vi "RS_Flip_Flop.vi"(3 "error in (no error)":errorcluster, 4 "Set":bool, 5 "Reset":bool) -> (0 "error out":errorcluster, 1 "Qnot":bool, 2 "Q":bool)   [LabVIEW 2018]
doc: "Set / Reset Flip Flop.\nR=0, S=0, Q=No change\nR=0, S=0, Q=1\nR=1, S=0, Q=0\nR=1, S=1, Q=invalid (will give an error)\n\nwritten by David Huff, DISTek Integration \n(www.distek.com)"
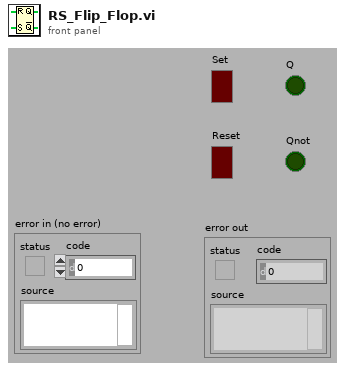
[diagram p1: front panel]
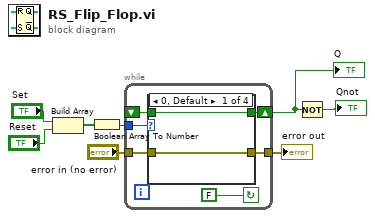
[diagram p0: block diagram]
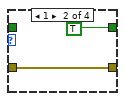
[diagram p2: hidden frame]
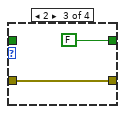
[diagram p3: hidden frame]
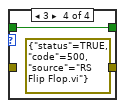
[diagram p4: hidden frame]
diagram:
  n1 = Build Array("Set", "Reset") -> (w6:bool[])
  n2 = Boolean Array To Number(Boolean array=w6) -> (number=w5:u32)
  n3 = while {
    shift-right: [w11] -> w4
    shift-left: _ -> [w12]
    tunnel: w5 -> [w13]
    tunnel: [w10] -> w2
    tunnel: "error in (no error)" -> [w9]
    stop <- FALSE continue-if-true
    n4 = case shown="0, Default" w13 {
      tunnel: [w16 TRUE FALSE w22] -> w11
      tunnel: w12 -> [w16 _ _ w22]
      tunnel: [w15 w17 w19 errorcluster {"status"=TRUE, "code"=500, "source"="RS Flip Flop.vi"} ("error in (no error)")] -> w10
      tunnel: w9 -> [w15 w17 w19 _]
      frame 0, Default {
      }
      frame 1 {
      }
      frame 2 {
      }
      frame 3 {
      }
    }
  }
  "error out" <- w2
  "Q" <- w4
  n5 = Not(x=w4) -> (.not. x?=→"Qnot":bool)
